vi "Overview Mouse Up.vi"(8 "error in":errorcluster, 11 "XYGraphOverview in":refnum<class "XYGraphOverview.lvclass">) -> (0 "error out":errorcluster, 3 "XYGraphOverview out":refnum<class "XYGraphOverview.lvclass">)   [LabVIEW 2020, in "XYGraphOverview.lvlib" / "XYGraphOverview.lvclass"]
uses:
  XYGraphOverview.lvclass
  XYGraphOverview.lvclass/XYGraphOverview.ctl
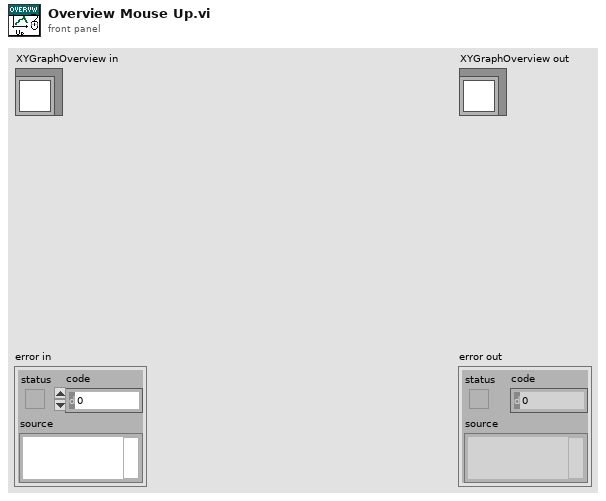
[diagram p1: front panel]
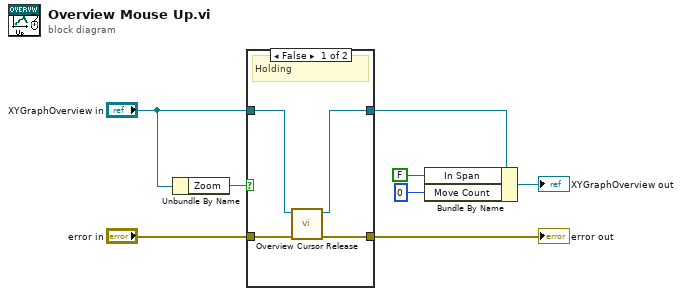
[diagram p0: block diagram]
diagram:
  n1 = Unbundle By Name("XYGraphOverview in") -> ("Zoom"=w2:bool)
  n2 = case shown="False" w2 {
    tunnel: [w11 w13] -> w8
    tunnel: "error in" -> [w10 w13]
    tunnel: [w9 w14] -> w7
    tunnel: "XYGraphOverview in" -> [w12 w14]
    frame False {
      # "Holding"
      n3 = call "Overview Cursor Release.vi"("error in"=w10, "XYGraphOverview in"=w12) -> ("error out"=w11:errorcluster, "XYGraphOverview out"=w9:refnum<class "XYGraphOverview.lvclass">)  [unwired: 8 in]
    }
    frame True {
      # "Fit"
    }
  }
  "error out" <- w8
  n4 = Bundle By Name(cluster=w7, "In Span"=FALSE, "Move Count"=u32 0) -> (→"XYGraphOverview out":refnum<class "XYGraphOverview.lvclass">)
